vi "Configure Diode.vi"(0 "VISA resource name":refnum<visa-resource-name>, 5 "error in (no error)":errorcluster, 8 "Range (0 A)":dbl format="%#_6p") -> (14 "VISA resource name out":refnum<visa-resource-name>, 19 "error out":errorcluster)   [LabVIEW 2021, in "Keithley 2000.lvlib"]
doc: "This VI configures the instrument to test a diode.\n\nNote:\nWhen reading measurements (using the \"Data Read Single\" or \"Data Read Multiple\" VIs), a value of 9.9E+37 indicates an open circuit. Any other value is the actual voltage."
uses:
  Keithley 2000.lvlib
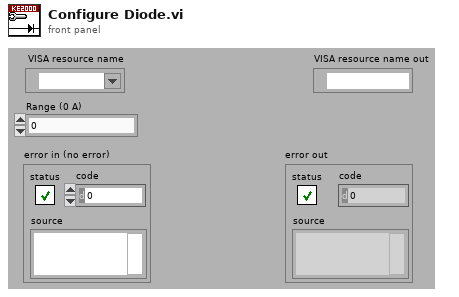
[diagram p1: front panel]
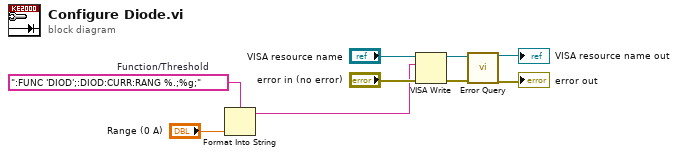
[diagram p0: block diagram]
diagram:
  w7 = ":FUNC 'DIOD';:DIOD:CURR:RANG %.;%g;"  # Function/Threshold
  n1 = Format Into String(format string=w7, "Range (0 A)") -> (resulting string=w5:string)  [unwired: 2 in, 1 out]
  n2 = VISA Write(VISA resource name="VISA resource name", write buffer=w5, error in (no error)="error in (no error)") -> (VISA resource name out=w4:refnum<visa-resource-name>, error out=w3:errorcluster)  [unwired: 1 out]
  n3 = call "Error Query.vi"("VISA resource name"=w4, "error in (no error)"=w3) -> ("VISA resource name out"=→"VISA resource name out":refnum<visa-resource-name>, "error out"=→"error out":errorcluster)  [unwired: 14 in, 2 out]
